vi "Release.vi"(8 "error in (no error)":errorcluster, 11 "Mapped Memory Access Image Greyscale":refnum<data-value>) -> (0 "error out":errorcluster, 3 "Greyscale Image":refnum<data-value>)   [LabVIEW 2020, in "g_ar_toolkit.image.lvlib" / "Mapped Memory Access Image Greyscale.lvclass"]
uses:
  Mapped Memory Access Image Greyscale.lvclass
  Mapped Memory Access Image Greyscale.lvclass/Mapped Memory Access Image Greyscale.ctl
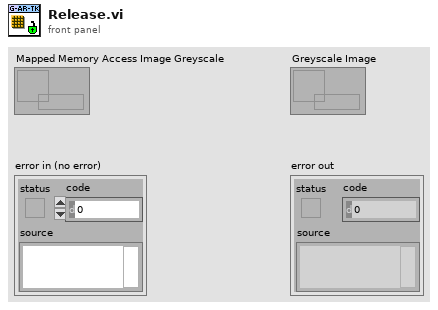
[diagram p1: front panel]
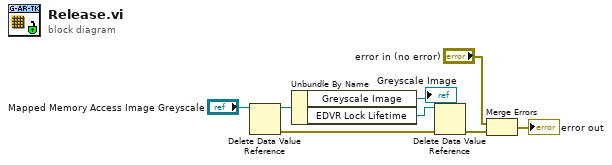
[diagram p0: block diagram]
diagram:
  n1 = Delete Data Value Reference(data value reference="Mapped Memory Access Image Greyscale") -> (data value=w6:refnum<class "Mapped Memory Access Image Greyscale.lvclass">, error out=w3:errorcluster)  [unwired: 1 in]
  n2 = Unbundle By Name(w6) -> ("Greyscale Image"=→"Greyscale Image":refnum<data-value>, "EDVR Lock Lifetime"=w4:refnum<data-value>)
  n3 = Delete Data Value Reference(data value reference=w4, error in=w3) -> (error out=w2:errorcluster)  [unwired: 1 out]
  n4 = Merge Errors("error in (no error)", w2) -> (→"error out":errorcluster)
